vi "globalTearDown.vi"(8 "error in (no error)":errorcluster, 11 "testcase-CSMSystemLevelModule in":refnum<class "testcase-CSMSystemLevelModule.lvclass">) -> (0 "error out":errorcluster, 3 "testcase-CSMSystemLevelModule out":refnum<class "testcase-CSMSystemLevelModule.lvclass">)   [LabVIEW 2017, in "testcase-CSMSystemLevelModule.lvclass"]
uses:
  testcase-CSMSystemLevelModule.lvclass
  testcase-CSMSystemLevelModule.lvclass/testcase-CSMSystemLevelModule.ctl
  <vilib>/addons/_JKI Toolkits/VI Tester/TestCase.llb/TestCase.lvclass
  src/user.lib/_NEVSTOP/Communicable State Machine(CSM)/_Support/Typedef/_CSM_List Module Scope.ctl
  src/user.lib/_NEVSTOP/Communicable State Machine(CSM)/Communicable State Machine.lvlib
panel:
  out "CSMs":string[](array[string])
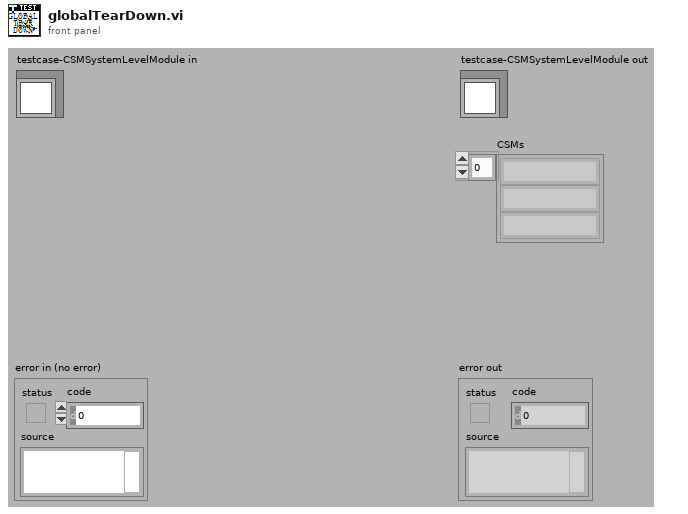
[diagram p1: front panel]
types:
  T1 = typedef "Communicable State Machine.lvlib/_CSM_List Module Scope.ctl" = enum16{"Normal", "System Only", "All"}
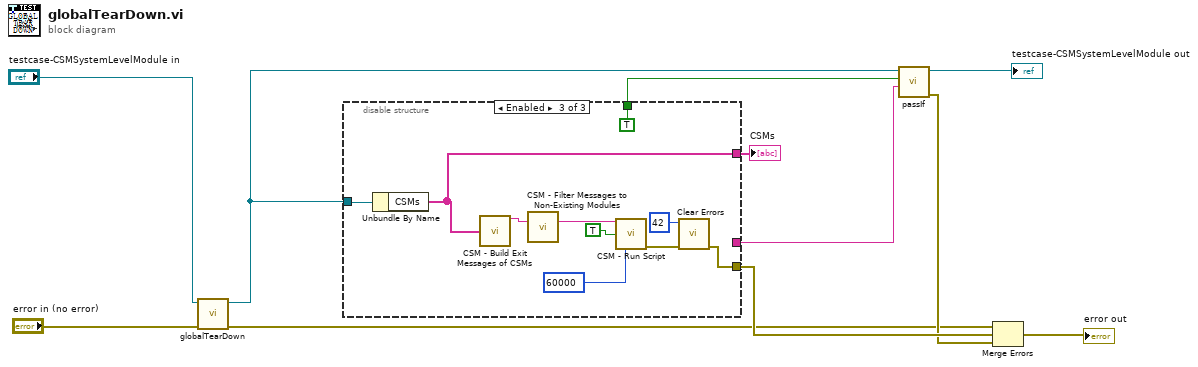
[diagram p0: block diagram]
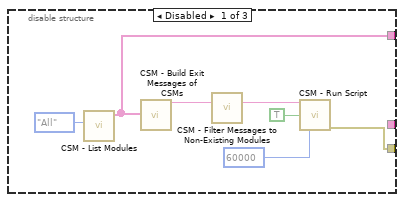
[diagram p2: hidden frame]
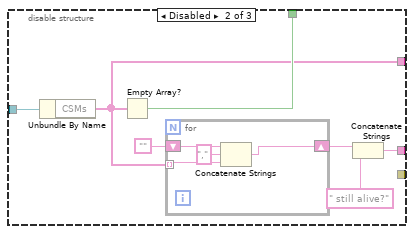
[diagram p3: hidden frame]
diagram:
  n1 = call-parent "globalTearDown.vi"("error in (no error)"="error in (no error)", "TestCase in"="testcase-CSMSystemLevelModule in") -> ("error out"=w5:errorcluster, "TestCase out"=w3:refnum<class "testcase-CSMSystemLevelModule.lvclass">)  [unwired: 8 in]
  n2 = disable-structure shown="Enabled" {
    disable-tunnel: [w14 _ w32] -> w7
    disable-tunnel: w3 -> [_ w25 w39]
    disable-tunnel: [w13 w23 w35] -> w1
    disable-tunnel: [_ w24 TRUE ("pass")] -> w9
    disable-tunnel: [_ w19 _] -> w8
    frame Disabled {
      n3 = call "CSM - List Modules.vi"("Scope (Normal)"=_CSM_List_Module_Scope."All") -> ("Module Names"=w13:string[])  [unwired: 9 in, 1 out]
      n4 = call "CSM - Build Exit Messages of CSMs.vi"("CSMs"=w13) -> ("States"=w18:string)  [unwired: 14 in]
      n5 = call "CSM - Filter Messages to Non-Existing Modules.vi"("States In"=w18) -> ("States Out"=w16:string)  [unwired: 14 in]
      n6 = call "CSM - Run Script.vi"("CSM Scripts"=w16, "Continue If Error? (F)"=TRUE, "Response Timeout (-2 Using Global Settings)"=60000) -> ("error out"=w14:errorcluster)  [unwired: 10 in, 2 out]
    }
    frame Disabled {
      n7 = Unbundle By Name(w25) -> ("CSMs"=w23:string[])
      n8 = Empty Array?(array=w23) -> (empty?=w24:bool)
      n9 = for {
        tunnel: w23 -> [w27] mode=indexing
        shift-right: [w28] -> w21
        shift-left: "" -> [w29]
        n10 = Concatenate Strings(w29, "," ("string"), w27) -> (w28:string)
      }
      n11 = Concatenate Strings(w21, " still alive?" ("string")) -> (w19:string)
    }
    frame Enabled {
      n12 = Unbundle By Name(w39) -> ("CSMs"=w35:string[])
      n13 = call "CSM - Build Exit Messages of CSMs.vi"("CSMs"=w35) -> ("States"=w38:string)  [unwired: 14 in]
      n14 = call "CSM - Filter Messages to Non-Existing Modules.vi"("States In"=w38) -> ("States Out"=w36:string)  [unwired: 14 in]
      n15 = call "CSM - Run Script.vi"("CSM Scripts"=w36, "Continue If Error? (F)"=TRUE, "Response Timeout (-2 Using Global Settings)"=60000) -> ("error out"=w34:errorcluster)  [unwired: 10 in, 2 out]
      n16 = call <vilib>:"Clear Errors.vi"("error in (no error)"=w34, "specific error code to clear (0: all)"=42) -> ("error out"=w32:errorcluster)  [unwired: 4 in, 1 out]
    }
  }
  "CSMs" <- w1
  n17 = call-dynamic "passIf.vi"("message (\"\")"=w8, "pass"=w9, "TestCase in"=w3) -> ("error out"=w6:errorcluster, "TestCase out"=→"testcase-CSMSystemLevelModule out":refnum<class "testcase-CSMSystemLevelModule.lvclass">)  [unwired: 7 in]
  n18 = Merge Errors(w5, w7, w6) -> (→"error out":errorcluster)
